vi "AT Centre AOI.vi"(8 "error in (no error)":errorcluster, 9 "AOI Width":i32, 10 "AOI Height":i32, 11 "Handle":i32) -> (0 "error out":errorcluster)   [LabVIEW 2019]
doc: "Centre AOI\n\nOutput:\n void\n\nInput:\n I32 Handle\n I64 AOI Height\n I64 AOI Width\n\nThis function will return the current value of the specified boolean feature. If a value of AT_FALSE is returned then the feature is currently set to false. If a value of AT_TRUE is returned then the feature is currently set to true. An error will be returned if the feature is currently not readable, not a boolean feature or is not implemented by the camera."
panel:
  in  "error":errorcluster
  out "Handle 2":i32
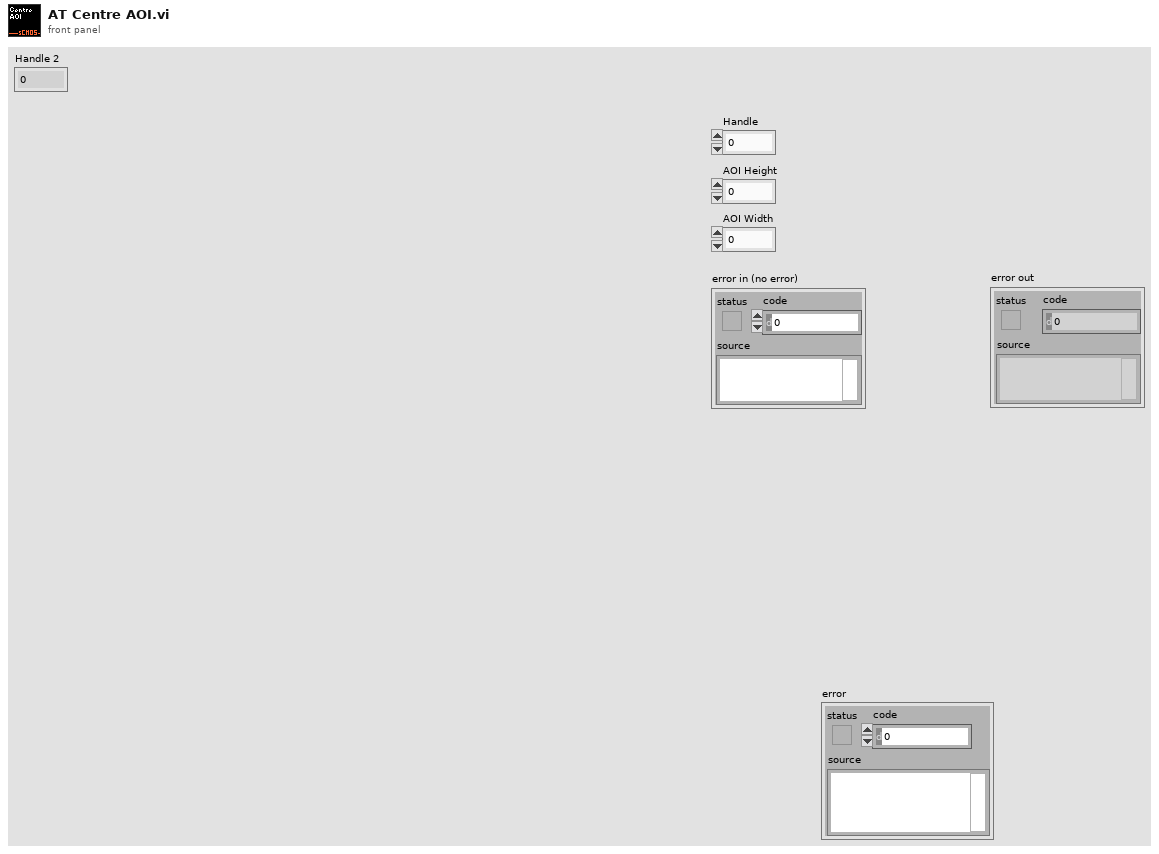
[diagram p1: front panel]
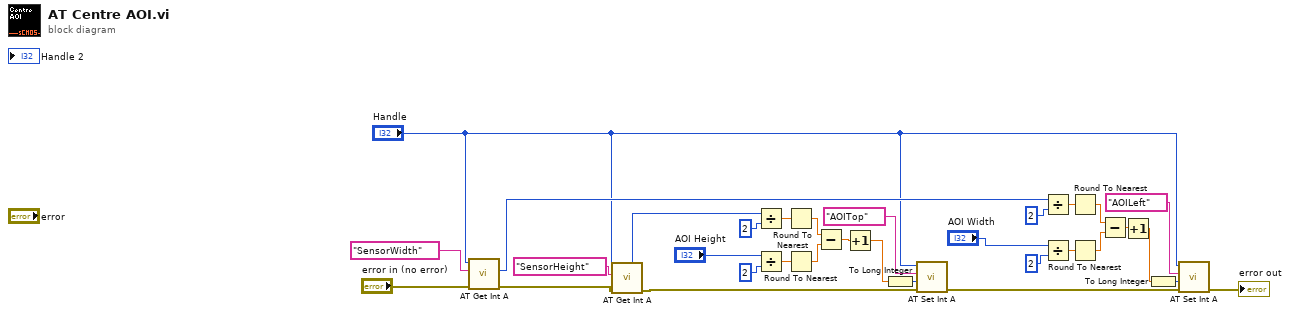
[diagram p0: block diagram]
diagram:
  n1 = call <userlib>:"AT Get Int A.vi"("error in (no error)"="error in (no error)", "Feature"="SensorWidth" ("Integer feature"), "Handle"="Handle") -> ("error out"=w10:errorcluster, "Value"=w15:i64)  [unwired: 6 in, 1 out]
  n2 = call <userlib>:"AT Get Int A.vi"("error in (no error)"=w10, "Feature"="SensorHeight" ("Integer feature"), "Handle"="Handle") -> ("error out"=w11:errorcluster, "Value"=w22:i64)  [unwired: 6 in, 1 out]
  n3 = Divide(x=w22, y=2) -> (x/y=w24:dbl)
  n4 = Divide(x="AOI Height", y=i64 2) -> (x/y=w29:dbl)
  n5 = Round To Nearest(number=w24) -> (nearest integer value=w25:dbl)
  n6 = Round To Nearest(number=w29) -> (nearest integer value=w28:dbl)
  n7 = Subtract(x=w25, y=w28) -> (x-y=w5:dbl)
  n8 = Increment(x=w5) -> (x+1=w4:dbl)
  n9 = To Long Integer(number=w4) -> (32bit integer=w13:i32)
  n10 = call <userlib>:"AT Set Int A.vi"("error in (no error)"=w11, "Value"=w13, "Feature"="AOITop" ("Integer feature 2"), "Handle"="Handle") -> ("error out"=w12:errorcluster)  [unwired: 6 in, 1 out]
  n11 = Divide(x=w15, y=i64 2) -> (x/y=w19:dbl)
  n12 = Divide(x="AOI Width", y=i64 2) -> (x/y=w18:dbl)
  n13 = Round To Nearest(number=w19) -> (nearest integer value=w21:dbl)
  n14 = Round To Nearest(number=w18) -> (nearest integer value=w20:dbl)
  n15 = Subtract(x=w21, y=w20) -> (x-y=w2:dbl)
  n16 = Increment(x=w2) -> (x+1=w3:dbl)
  n17 = To Long Integer(number=w3) -> (32bit integer=w14:i32)
  n18 = call <userlib>:"AT Set Int A.vi"("error in (no error)"=w12, "Value"=w14, "Feature"="AOILeft" ("Integer feature"), "Handle"="Handle") -> ("error out"=→"error out":errorcluster)  [unwired: 6 in, 1 out]
